vi "Elasped_Time.vi"() -> ()   [LabVIEW 2019]
panel:
  in  "stop":bool
  in  "Reset":bool
  in  "Time Target (s)":dbl=10.0
  out "error out":errorcluster
  in  "error in (no error)":errorcluster
  out "Boolean":bool
  out "Elapsed Time (s)":dbl
  out "Present (s)":dbl
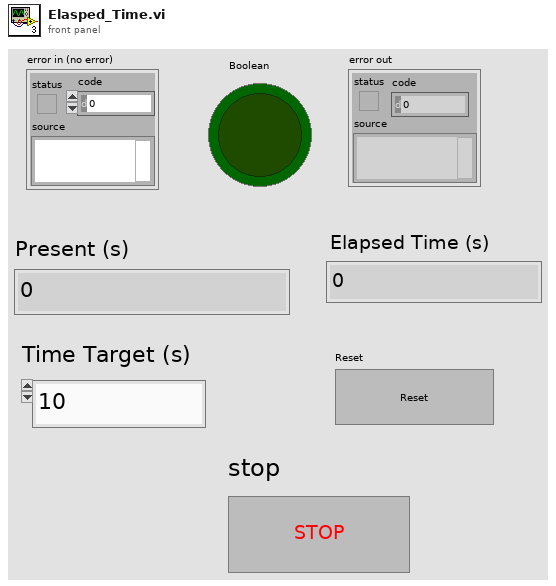
[diagram p1: front panel]
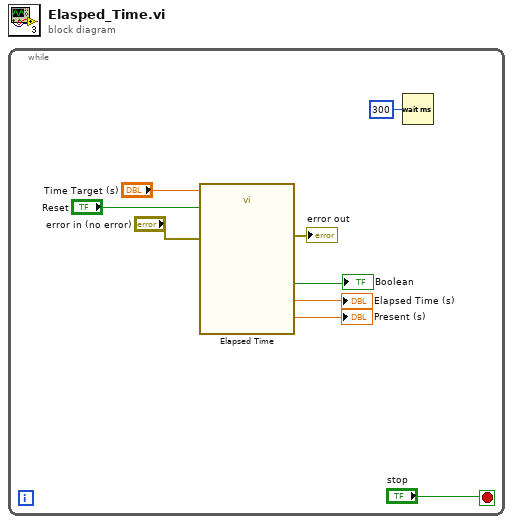
[diagram p0: block diagram]
diagram:
  n1 = while {
    stop <- "stop" stop-if-true
    n2 = call "Elapsed Time"("Time Target (s)"="Time Target (s)", "Reset"="Reset", "error in (no error)"="error in (no error)") -> ("Present (s)"=→"Present (s)":dbl, "Elapsed Time (s)"=→"Elapsed Time (s)":dbl, "Time has Elapsed"=→"Boolean":bool, "error out"=→"error out":errorcluster)  [unwired: 9 in, 4 out]
    n3 = Wait (ms)(milliseconds to wait=u32 300) -> ()  [unwired: 1 out]
  }
